vi "Configure Digital Burst.vi"(6 "Burst Period (.001 s)":dbl=0.001, 7 "Burst Mode (0: bmNone)":i32(ring) items=["bmNone", "bmTimed"], 8 "error in (no error)":errorcluster, 9 "Low Amplitude (0.0 %)":dbl, 10 "Duty Cycle (.50 %)":dbl=0.5, 11 "VISA resource name":refnum<visa-resource-name>) -> (0 "error out":errorcluster, 3 "VISA resource name out":refnum<visa-resource-name>)   [LabVIEW 2014, in "Stanford Research SR1.lvlib"]
doc: "Configures the attributes for the Digital Burst."
uses:
  Stanford Research SR1.lvlib
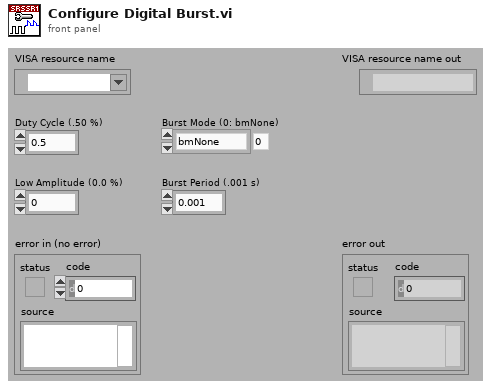
[diagram p1: front panel]
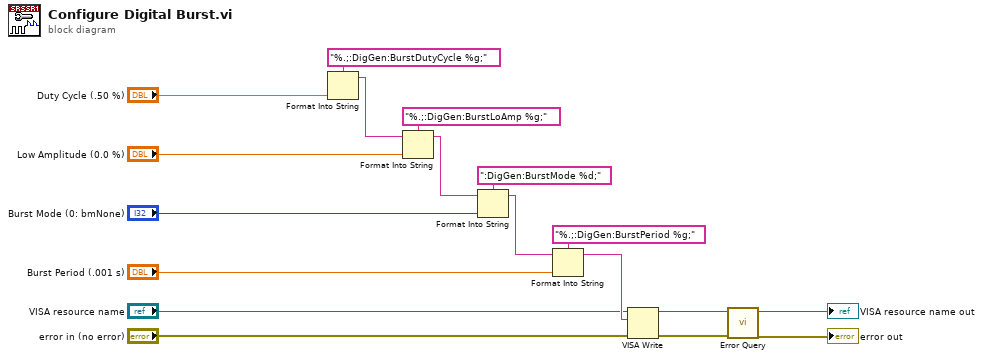
[diagram p0: block diagram]
diagram:
  n1 = Format Into String(format string="%.;:DigGen:BurstDutyCycle %g;", "Duty Cycle (.50 %)") -> (resulting string=w16:string)  [unwired: 2 in, 1 out]
  n2 = Format Into String(format string="%.;:DigGen:BurstLoAmp %g;", initial string=w16, "Low Amplitude (0.0 %)") -> (resulting string=w13:string)  [unwired: 1 in, 1 out]
  n3 = Format Into String(format string=":DigGen:BurstMode %d;", initial string=w13, "Burst Mode (0: bmNone)") -> (resulting string=w10:string)  [unwired: 1 in, 1 out]
  n4 = Format Into String(format string="%.;:DigGen:BurstPeriod %g;", initial string=w10, "Burst Period (.001 s)") -> (resulting string=w7:string)  [unwired: 1 in, 1 out]
  n5 = VISA Write(VISA resource name="VISA resource name", write buffer=w7, error in (no error)="error in (no error)") -> (VISA resource name out=w4:refnum<visa-resource-name>, error out=w3:errorcluster)  [unwired: 1 out]
  n6 = call "Error Query.vi"("error in (no error)"=w3, "VISA resource name"=w4) -> ("error out"=→"error out":errorcluster, "VISA resource name out"=→"VISA resource name out":refnum<visa-resource-name>)  [unwired: 6 in, 2 out]
